vi "SetChannelRequest.vi"(8 "error in (no error)":errorcluster, 10 "Channels":T1, 11 "ModuleID":i32) -> (0 "error out":errorcluster)   [LabVIEW 2018, in "ScopeModule.lvlib"]
uses:
  ScopeModule.lvlib
  ScopeShared/clEventType.ctl
  <vilib>/Utility/error.llb/Error Cluster From Error Code.vi
  <vilib>/ErrorRing/Error Ring.xnode
  ScopeShared/ScopeShared.lvlib
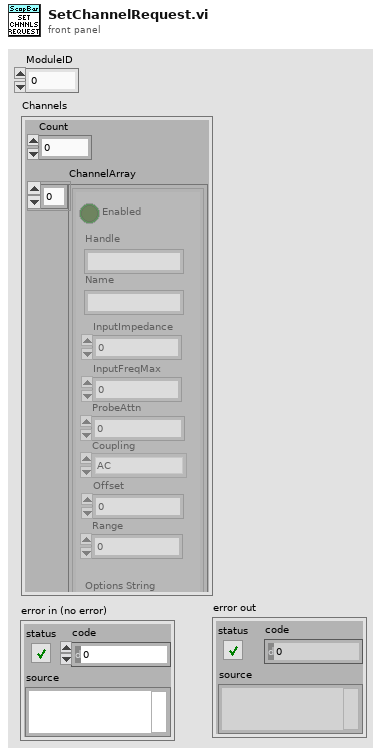
[diagram p1: front panel]
types:
  T1 = cluster{"Count":i32, "ChannelArray":cluster{"Enabled":bool, "Name":string, "InputImpedance":dbl, "InputFreqMax":dbl, "ProbeAttn":dbl, "Coupling":enum16{"AC", "DC", "GND"}, "Offset":dbl, "Range":dbl, "Handle":string, "Connected":bool, "Options String ":string}[]}
  T2 = typedef "ScopeShared.lvlib/clRequestEvents.ctl" = cluster{"StopRequest":refnum<user-event>, "PathToINI":refnum<user-event>, " LoadPlugin":refnum<user-event>, "ShowPanel":refnum<user-event>, "Abort":refnum<user-event>, "SetAcquisition":refnum<user-event>, "SetChannel":refnum<user-event>, "SetTrigger":refnum<user-event>, "GetAcquisition":refnum<user-event>, "GetChannel":refnum<user-event>, "GetTrigger":refnum<user-event>, "FetchWaveform":refnum<user-event>, "InitAcquisition":refnum<user-event>, "ReadWaveform":refnum<user-event>, "GetHandle":refnum<user-event>, "SetHandle":refnum<user-event>, "GetModel":refnum<user-event>, "SetModel":refnum<user-event>, "ConfigAquisition":refnum<user-event>, "ConfigChannels":refnum<user-event>, "ConfigTrigger":refnum<user-event>, "Initialize":refnum<user-event>, "SetExtAcquisition":refnum<user-event>, "StopAcquisition":refnum<user-event>, "PrefDlg":refnum<user-event>, "Close":refnum<user-event>, "SetSync":refnum<user-event>}
  T3 = typedef "ScopeShared.lvlib/clEventType.ctl" = cluster{"ModuleID":i32, "Data":variant}
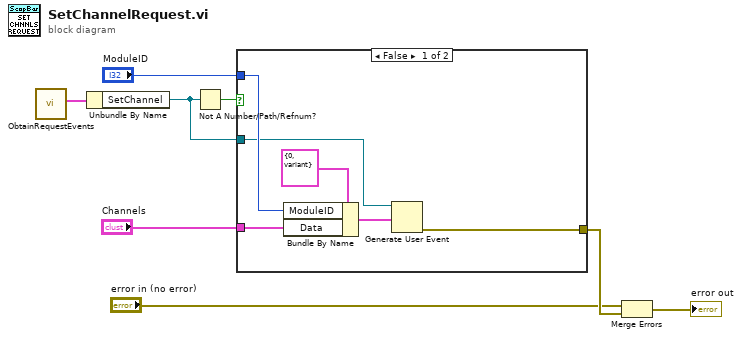
[diagram p0: block diagram]
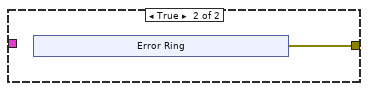
[diagram p2: hidden frame]
diagram:
  n1 = call "ObtainRequestEvents.vi"() -> ("ScopeRequests"=w8:T2)  [unwired: 10 in, 1 out]
  n2 = Unbundle By Name(w8) -> ("SetChannel"=w6:refnum<user-event>)
  n3 = Not A Number/Path/Refnum?(number/path/refnum=w6) -> (NaN/Path/Refnum?=w7:bool)
  n4 = case shown="False" w7 {
    tunnel: w6 -> [w11 _]
    tunnel: "ModuleID" -> [w13 _]
    tunnel: [w10 w15] -> w3
    tunnel: "Channels" -> [w9 _]
    frame False {
      n5 = Bundle By Name(cluster=T3 {"ModuleID"=0, "Data"=variant} ("clEventType"), "ModuleID"=w13, "Data"=w9) -> (w12:T3)
      n6 = Generate User Event(user event=w11, event data cluster=w12) -> (error out=w10:errorcluster)  [unwired: 2 in, 1 out]
    }
    frame True {
      n7 = xnode "Error Ring"() -> ("error out"=w15:errorcluster)
    }
  }
  n8 = Merge Errors("error in (no error)", w3) -> (→"error out":errorcluster)
